vi "VMI_move_PI.vi"(7 "Delay Cluster":T1={"System no."=0, "Identification"="", "Device ID out"=0, "Postion / mm"=[], "SN out"="", "Movement Range"=[], "Conn. Axes"=[], "Target Position / mm"=50.0, "Velocity / mm s^-1"=0.15, "Set-up"=FALSE, "Moving"=FALSE, "Step Size / mm "=0.15, "Stage Number"=0, "Polling Time /ms"=0}, 8 "Error In":errorcluster, 10 "Stop ref":refnum<vi>, 11 "position ref":refnum<vi>) -> (0 "error out":errorcluster)   [LabVIEW 2015]
uses:
  Type defs/PI_delay_settings.ctl
panel:
  in  "Stop Button":bool
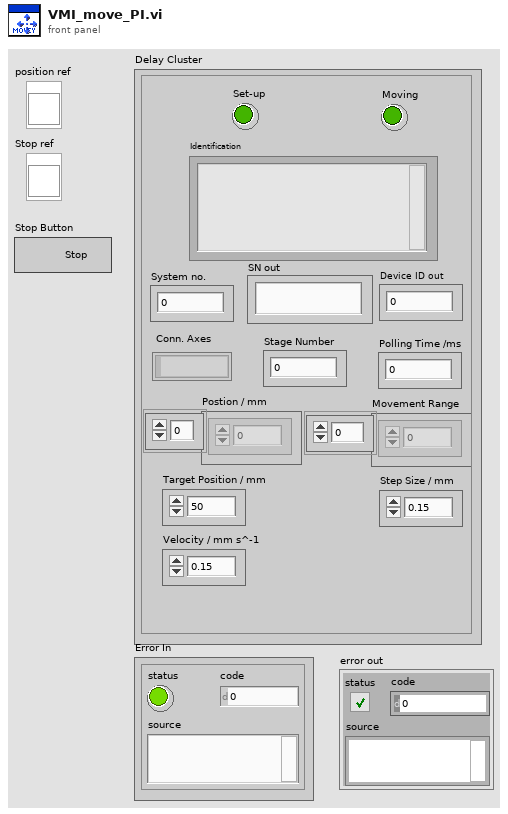
[diagram p1: front panel]
types:
  T1 = typedef "PI_delay_settings.ctl" = cluster{"System no.":i32, "Identification":string, "Device ID out":i32, "Postion / mm":dbl[], "SN out":string, "Movement Range":dbl[], "Conn. Axes":string[], "Target Position / mm":dbl, "Velocity / mm s^-1":dbl, "Set-up":bool, "Moving":bool, "Step Size / mm ":dbl, "Stage Number":i32, "Polling Time /ms":i32}
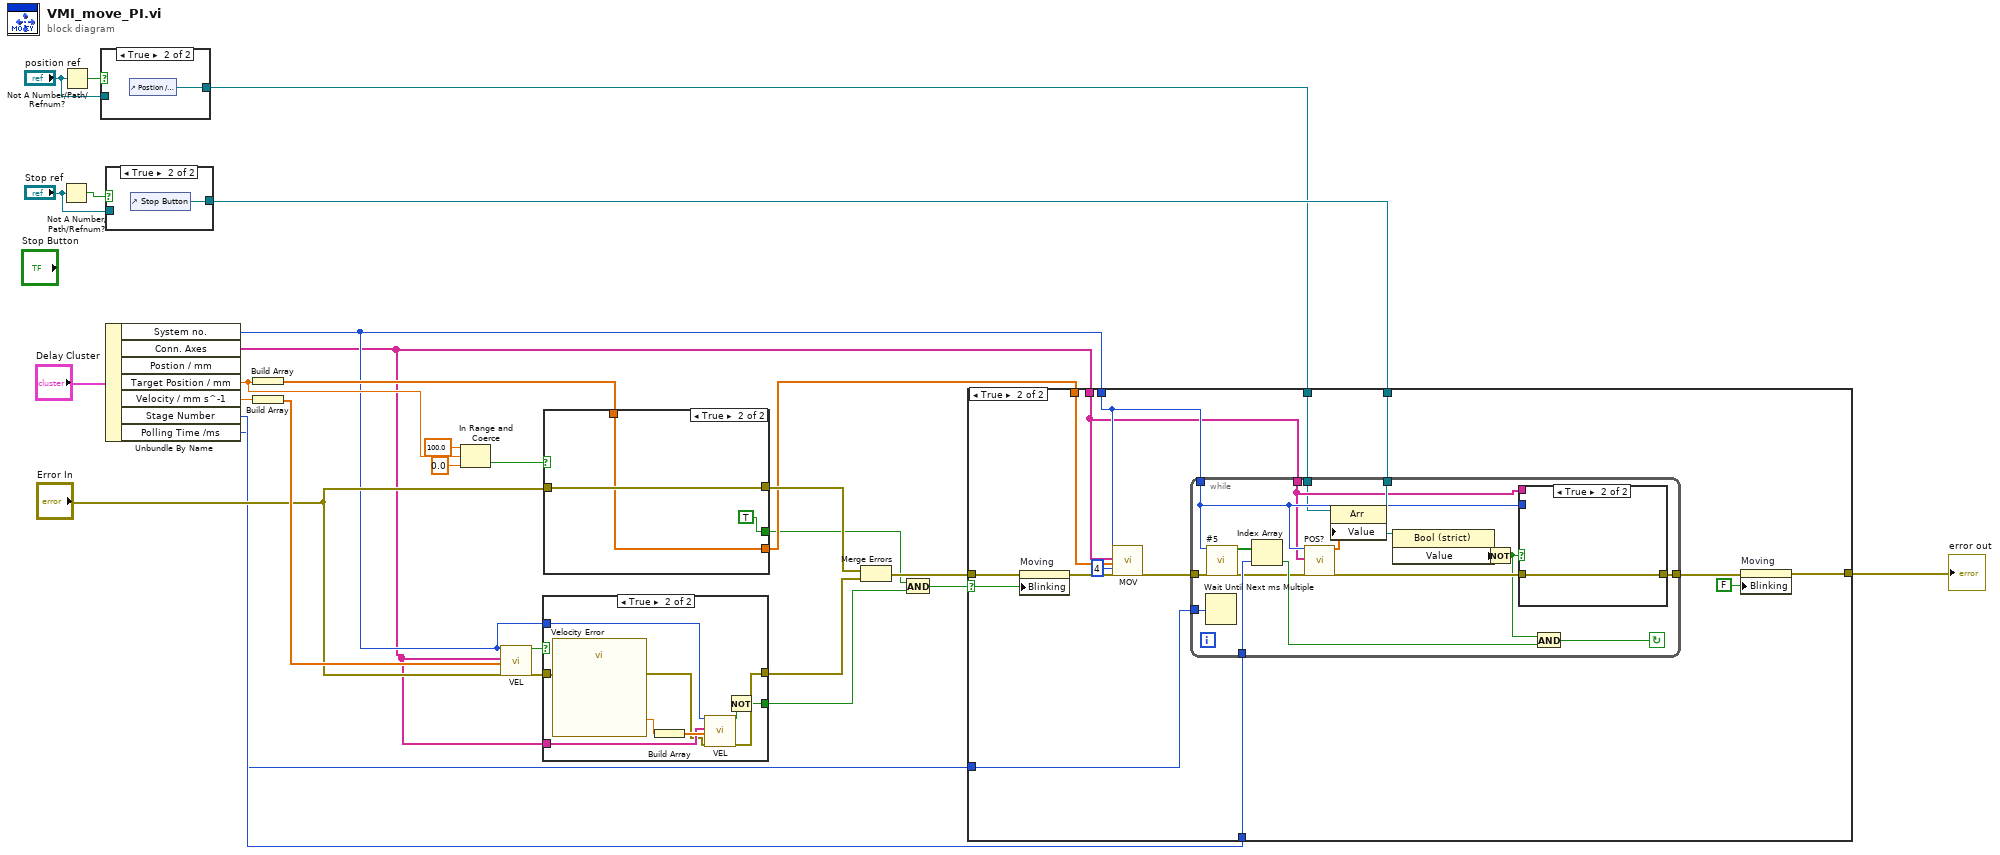
[diagram p0: block diagram]
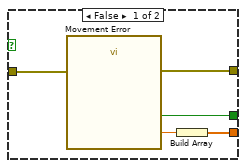
[diagram p4: hidden frame]
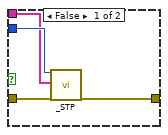
[diagram p6: hidden frame]
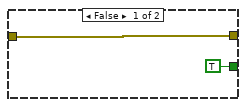
[diagram p7: hidden frame]
diagram:
  n1 = Not A Number/Path/Refnum?(number/path/refnum="Stop ref") -> (NaN/Path/Refnum?=w11:bool)
  n2 = Not A Number/Path/Refnum?(number/path/refnum="position ref") -> (NaN/Path/Refnum?=w4:bool)
  n3 = case shown="True" w4 {
    tunnel: [w30 w31] -> w3
    tunnel: "position ref" -> [w30 _]
    frame False {
    }
    frame True {
      n4 = control-ref of="Postion / mm"() -> (w31:refnum<vi>)
    }
  }
  n5 = case shown="True" w11 {
    tunnel: [w32 w33] -> w9
    tunnel: "Stop ref" -> [w32 _]
    frame False {
    }
    frame True {
      n6 = control-ref of="Stop Button"() -> (w33:refnum<vi>)
    }
  }
  n7 = Unbundle By Name("Delay Cluster") -> ("System no."=w8:i32, "Conn. Axes"=w7:string[], "Target Position / mm"=w17:dbl, "Velocity / mm s^-1"=w28:dbl, "Stage Number"=w2:i32, "Polling Time /ms"=w1:i32)  [unwired: 1 out]
  n8 = Build Array(w17) -> (w20:dbl[])
  n9 = Build Array(w28) -> (w27:dbl[])
  n10 = In Range and Coerce(upper limit=100.0, x=w17, lower limit=0.0) -> (In Range?=w15:bool)  [unwired: 1 out]
  n11 = call "VEL.vi"("System no."=w8, "Axes to set"=w7, "Velocity values"=w27, "error in"="Error In") -> ("Controller error"=w26:bool, "error out"=w25:errorcluster)  [unwired: 2 in, 12 out]
  n12 = case shown="True" w26 {
    tunnel: w25 -> [w35 w44]
    tunnel: [w35 w38] -> w22
    tunnel: [TRUE ("OK") w36] -> w14
    tunnel: w8 -> [_ w41]
    tunnel: w7 -> [_ w40]
    frame False {
    }
    frame True {
      n13 = call "Velocity Error"("error in (no error)"=w44) -> ("Velocity"=w43:dbl, "error out"=w39:errorcluster)  [unwired: 16 in, 1 out]
      n14 = Build Array(w43) -> (w42:dbl[])
      n15 = call "VEL.vi"("System no."=w41, "Axes to set"=w40, "Velocity values"=w42, "error in"=w39) -> ("Controller error"=w37:bool, "error out"=w38:errorcluster)  [unwired: 2 in, 12 out]
      n16 = Not(x=w37) -> (.not. x?=w36:bool)
    }
  }
  n17 = case shown="True" w15 {
    tunnel: "Error In" -> [w49 w52]
    tunnel: [w48 w52] -> w23
    tunnel: [w47 TRUE ("OK")] -> w12
    tunnel: [w45 w50] -> w19
    tunnel: w20 -> [_ w50]
    frame False {
      n18 = call "Movement Error"("error in (no error)"=w49) -> ("Target"=w46:dbl, "OK"=w47:bool, "error out"=w48:errorcluster)  [unwired: 16 in]
      n19 = Build Array(w46) -> (w45:dbl[])
    }
    frame True {
    }
  }
  n20 = Merge Errors(w23, w22) -> (w21:errorcluster)
  n21 = And(x=w12, y=w14) -> (x .and. y?=w13:bool)
  n22 = case shown="True" w13 {
    selector: w13 -> [_ w65]
    tunnel: w19 -> [_ w68]
    tunnel: w8 -> [_ w61]
    tunnel: w7 -> [_ w59]
    tunnel: w21 -> [w53 w66]
    tunnel: [w53 w63] -> w6
    tunnel: w2 -> [_ w60]
    tunnel: w9 -> [_ w56]
    tunnel: w3 -> [_ w55]
    tunnel: w1 -> [_ w54]
    frame False {
    }
    frame True {
      n23 = property on="Moving" class="Bool (strict)"(error in=w66, "Blinking"=w65) -> (error out=w64:errorcluster)  [unwired: 1 in, 1 out]
      n24 = call "MOV.vi"("System no."=w61, "Axes to move"=w59, "Position values"=w68, "No.of digits"=i16 4, "error in"=w64) -> ("error out"=w62:errorcluster)  [unwired: 14 out]
      n25 = while {
        tunnel: w62 -> [w84]
        tunnel: w61 -> [w71]
        tunnel: w60 -> [w82]
        tunnel: w59 -> [w70]
        tunnel: [w74] -> w58
        tunnel: w54 -> [w78]
        tunnel: w56 -> [w77]
        tunnel: w55 -> [w69]
        stop <- w73 continue-if-true
        n26 = Wait Until Next ms Multiple(millisecond multiple=w78) -> ()  [unwired: 1 out]
        n27 = call "#5.vi"("System no."=w71, "error in"=w84) -> ("Axis moving?"=w83:bool[], "error out"=w80:errorcluster)  [unwired: 16 in]
        n28 = Index Array(array=w83, index=w82) -> (element=w81:bool)
        n29 = call "POS?.vi"("System no."=w71, "Axes to query"=w70, "error in"=w80) -> ("Position"=w79:dbl[], "error out"=w75:errorcluster)  [unwired: 15 in]
        n30 = property on="Property Node" class="Arr"(reference=w69, "Value"=w79) -> ()  [unwired: 1 in, 2 out]
        n31 = property class="Bool (strict)"(reference=w77) -> ("Value"=w76:bool)  [unwired: 1 in, 2 out]
        n32 = Not(x=w76) -> (.not. x?=w72:bool)
        n33 = case shown="True" w72 {
          tunnel: w75 -> [w88 w89]
          tunnel: [w87 w89] -> w74
          tunnel: w71 -> [w86 _]
          tunnel: w70 -> [w85 _]
          frame False {
            n34 = call "_STP.vi"("System no."=w86, "Affected axes?"=w85, "error in"=w88) -> ("error out"=w87:errorcluster)  [unwired: 16 in]
          }
          frame True {
          }
        }
        n35 = And(x=w72, y=w81) -> (x .and. y?=w73:bool)
      }
      n36 = property on="Moving" class="Bool (strict)"(error in=w58, "Blinking"=FALSE) -> (error out=w63:errorcluster)  [unwired: 1 in, 1 out]
    }
  }
  "error out" <- w6
